vi "Get Position Achieved.vi"(4 "error in (no error)":errorcluster, 6 "Axis In":i16, 7 "Controller Reference In":refnum<k7>) -> (0 "error out":errorcluster, 1 "PosAchieved":bool, 2 "Axis Out":i16, 3 "Controller Reference Out":refnum<k7>)   [LabVIEW 2015]
doc: "Checks if the desired position has been acheived by the axis."
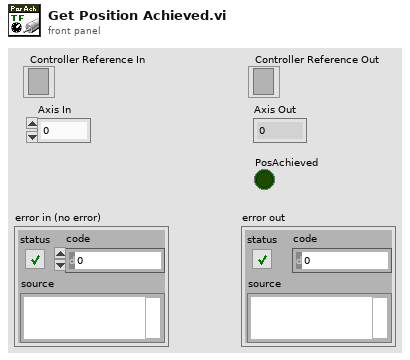
[diagram p1: front panel]
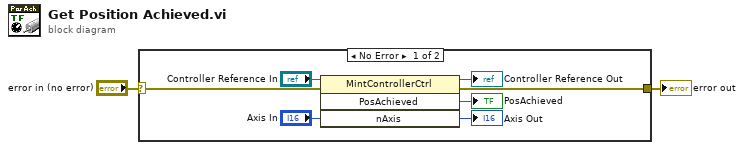
[diagram p0: block diagram]
diagram:
  n1 = case shown="No Error" "error in (no error)" {
    selector: "error in (no error)" -> [w4 w10]
    tunnel: [w7 w10] -> w2
    frame No Error {
      n2 = invoke class="MintControllerCtrl" method="PosAchieved"(reference="Controller Reference In", error in=w4, "nAxis"="Axis In") -> (reference out=→"Controller Reference Out":refnum<k7>, error out=w7:errorcluster, "PosAchieved"=→"PosAchieved":bool, "nAxis"=→"Axis Out":i16)  [unwired: 1 in]
    }
    frame Error {
    }
  }
  "error out" <- w2
